vi "FG_Messen.vi"(0 "Peiker_Stepped Sweep Settings":T5={"Input Settings"={"IEPE min time to settle [s]"=0.0, "Responce Channel Settings"={"DSA response channel settings"={"coupling"=10045, "enable IEPE excitation"=FALSE, "IEPE current [mA]"=4.0}, "response channel info"={"sensor sensitivity"=1000.0, "engineering units"=1, "dB reference"=1.0, "custom label"="EU", "weighting filter"=0, "pregain"=0.0}, "AI response settings"={"response channel"="SOUNDACQ/ai1", "max value [V]"=10.0, "min value [V]"=-10.0, "terminal configuration"=-1}}, "Stimulus Channel Settings"={"AI stimulus settings"={"stimulus channel"="SOUNDACQ/ai0", "max value [V]"=2.0, "min value [V]"=-2.0, "terminal configuration"=-1}, "DSA stimulus channel settings"={"coupling"=10045, "enable IEPE excitation"=TRUE, "IEPE current [mA]"=4.0}, "stimulus channel info"={"sensor sensitivity"=11.4, "engineering units"=2, "dB reference"=2e-05, "custom label"="EU", "weighting filter"=0, "pregain"=0.0}}}, "Output Settings"={"AO source settings"={"excitation channel"="SOUNDACQ/ao0", "max value [V]"=10.0, "min value [V]"=-10.0, "terminal configuration"=-1}}} {"Output Settings"."AO source settings"."terminal configuration" items=["Default"=-1, "RSE"=10083, "Differential"=10106, "Pseudodifferential"=12529]; "Output Settings"."AO source settings"."min value [V]" format="%0.2f"; "Output Settings"."AO source settings"."max value [V]" format="%0.2f"; "Input Settings"."Stimulus Channel Settings"."stimulus channel info"."pregain" format="%.2f"; "Input Settings"."Stimulus Channel Settings"."stimulus channel info"."weighting filter" items=["Linear", "A-weighting", "B-weighting", "C-weighting", "ITU-R 468-4", "Dolby", "CCITT", "C-message", "Wb", "Wc", "Wd", "We", "Wf", "Wh", "Wj", "Wk", "Wm", "AES17 20 kHz lowpass", "AES17 40 kHz lowpass", "AES17 20 kHz highpass", "AES17 40 kHz highpass"]; "Input Settings"."Stimulus Channel Settings"."stimulus channel info"."dB reference" format="%^.1e"; "Input Settings"."Stimulus Channel Settings"."stimulus channel info"."engineering units" items=["custom..."=0, "V"=1, "A"=21, "C"=30, "pC"=31, "s"=32, "-"=29, "Pa"=2, "N"=20, "g"=3, "m/s^2"=4, "m/s"=5, "m"=6, "mm/s"=12, "mm"=13, "micron/s"=14, "micron"=15, "in/s^2"=7, "in/s"=8, "in"=9, "mil/s"=10, "mil"=11, "rad/s^2"=16, "rad/s"=17, "rad"=18, "deg/s^2"=26, "deg/s"=27, "deg"=28, "RPM"=22, "cycle/s^2"=23, "Hz"=24, "cycle"=25, "strain"=19]; "Input Settings"."Stimulus Channel Settings"."stimulus channel info"."sensor sensitivity" format="%#_5f"; "Input Settings"."Stimulus Channel Settings"."DSA stimulus channel settings"."IEPE current [mA]" format="%.1f"; "Input Settings"."Stimulus Channel Settings"."DSA stimulus channel settings"."coupling" items=["AC"=10045, "DC"=10050, "GND"=10066]; "Input Settings"."Stimulus Channel Settings"."AI stimulus settings"."terminal configuration" items=["Default"=-1, "RSE"=10083, "NRSE"=10078, "Differential"=10106, "Pseudodifferential"=12529]; "Input Settings"."Stimulus Channel Settings"."AI stimulus settings"."min value [V]" format="%.2f"; "Input Settings"."Stimulus Channel Settings"."AI stimulus settings"."max value [V]" format="%.2f"; "Input Settings"."Responce Channel Settings"."AI response settings"."terminal configuration" items=["Default"=-1, "RSE"=10083, "NRSE"=10078, "Differential"=10106, "Pseudodifferential"=12529]; "Input Settings"."Responce Channel Settings"."AI response settings"."min value [V]" format="%.2f"; "Input Settings"."Responce Channel Settings"."AI response settings"."max value [V]" format="%.2f"; "Input Settings"."Responce Channel Settings"."response channel info"."pregain" format="%.2f"; "Input Settings"."Responce Channel Settings"."response channel info"."weighting filter" items=["Linear", "A-weighting", "B-weighting", "C-weighting", "ITU-R 468-4", "Dolby", "CCITT", "C-message", "Wb", "Wc", "Wd", "We", "Wf", "Wh", "Wj", "Wk", "Wm", "AES17 20 kHz lowpass", "AES17 40 kHz lowpass", "AES17 20 kHz highpass", "AES17 40 kHz highpass"]; "Input Settings"."Responce Channel Settings"."response channel info"."dB reference" format="%^.1e"; "Input Settings"."Responce Channel Settings"."response channel info"."engineering units" items=["custom..."=0, "V"=1, "A"=21, "C"=30, "pC"=31, "s"=32, "-"=29, "Pa"=2, "N"=20, "g"=3, "m/s^2"=4, "m/s"=5, "m"=6, "mm/s"=12, "mm"=13, "micron/s"=14, "micron"=15, "in/s^2"=7, "in/s"=8, "in"=9, "mil/s"=10, "mil"=11, "rad/s^2"=16, "rad/s"=17, "rad"=18, "deg/s^2"=26, "deg/s"=27, "deg"=28, "RPM"=22, "cycle/s^2"=23, "Hz"=24, "cycle"=25, "strain"=19]; "Input Settings"."Responce Channel Settings"."response channel info"."sensor sensitivity" format="%#_5f"; "Input Settings"."Responce Channel Settings"."DSA response channel settings"."IEPE current [mA]" format="%.1f"; "Input Settings"."Responce Channel Settings"."DSA response channel settings"."coupling" items=["AC"=10045, "DC"=10050, "GND"=10066]; "Input Settings"."IEPE min time to settle [s]" format="%.1f"}, 1 "settling time":T11={"settle time [s]"=0.03, "settle cycles"=5} {"settle time [s]" format="%.2p"}, 2 "FrequencyList Output Level (dBSPL)":dbl=94.0, 5 "frequency list Input":T4(array[cluster])=[{"frequency [Hz]"=103.0, "amplitude [V]"=0.09342446715491094}] {"amplitude [V]" format="%.6f"; "frequency [Hz]" format="%.2f"}, 9 "true=mehrfach Messen":bool, 11 "error in (no error)":errorcluster, 12 "FrequencyList Input Level (dBSPL)":dbl=94.0, 13 "integration time":T10={"integration time [s]"=0.03, "integration cycles"=5} {"integration cycles" min=2; "integration time [s]" format="%.2p"}) -> (3 "Fundamental-Response":T1(graph), 4 "THD-Response":cluster{"frequency":dbl[], "THD":dbl[]}(graph), 6 "Harmonics-Response":cluster{"frequency":dbl[], "distortion":dbl[]}[](graph), 8 "Fundamental-Response dB berechnet":T3(graph) caption="Fundamental-Response dB berechnet aus THD-Modul", 10 "fundamental amplitude":T1, 14 "Stimulus Level":cluster{"frequency":dbl[], "magnitude":dbl[]}(graph), 15 "error out":errorcluster={"status"=FALSE, "code"=0, "source"="\r\n"})   [LabVIEW 2018]
doc: "Das VI dient dem Messen eines Frequenzgangs. \nDieser kann verwendet werden um den Speaker abzugleichen.\nEin abweichender Pegel darf erst angegeben werden, wenn ein Speakerabgleich auf 94 dBSpl erfolgt ist.\n\nDie 94dB Spannungswerte werden dann auf den gewünschten Pegel umgerechnet."
uses:
  Peiker_Stepped Sweep Settings.ctl
  <vilib>/addons/_NISVFA/_Shared subVIs/Controls/svc_DSA Channel Settings.ctl
  <vilib>/addons/_NISVFA/_Shared subVIs/Controls/svc_Channel Info.ctl
  <vilib>/addons/_NISVFA/_Shared subVIs/Controls/svc_Engineering Units Text Ring.ctl
  <vilib>/addons/_NISVFA/_Shared subVIs/Controls/svc_Weighting Filter Text Ring.ctl
  <vilib>/addons/Sound and Vibration/svt_Swept Sine/SVT Initialize Swept Sine (DAQmx) (1 AO, 2 AI).vi
  <vilib>/addons/_NISVFA/_Baseband FFT/SVFA Power Spectrum (N Ch).vi
  <vilib>/addons/Sound and Vibration/svt_Swept Sine/SoundVib_SweptSine.lvlib
panel:
  out "Waveform Graph 4":waveform(dbl)[](graph)
  in  "Tab Control":T2(tab)
  out "Waveform Graph 2":waveform(dbl)[](graph)
  in  "Messkurve":dbl min=0.0 max=28.0
  out "Block Duration":waveform(dbl)[](graph)
  in  "stop":bool
  in  "Enable this Diagramm":bool
  out "Waveform Graph 3":cluster{"f0":dbl, "df":dbl, "magnitude":dbl[]}[](graph)
  out "Response Level":cluster{"frequency":dbl[], "magnitude":dbl[]}(graph)
  out "THD":cluster{"frequency":dbl[], "THD":dbl[]}={"frequency"=[103.0], "THD"=[0.2630754420190896]} {"THD" format="%.2f"; "frequency" format="%.2f"}
  out "Waveform Graph":cluster{"f0":dbl, "df":dbl, "magnitude":dbl[]}[](graph)
  out "FrequencyList Output Level":T4(graph)
  in  "Anzahl der Messungen bei einer Frequenz":i32=10
  in  "block duration [ms]":dbl=30.0
  in  "sample rate [Hz]":dbl=50000.0
  out "status":T12 {"% complete" format="%.2f"; "current processed frequency" format="%.2f"; "current source frequency" format="%.2f"; "elapsed time [s]" format="%.2f"}
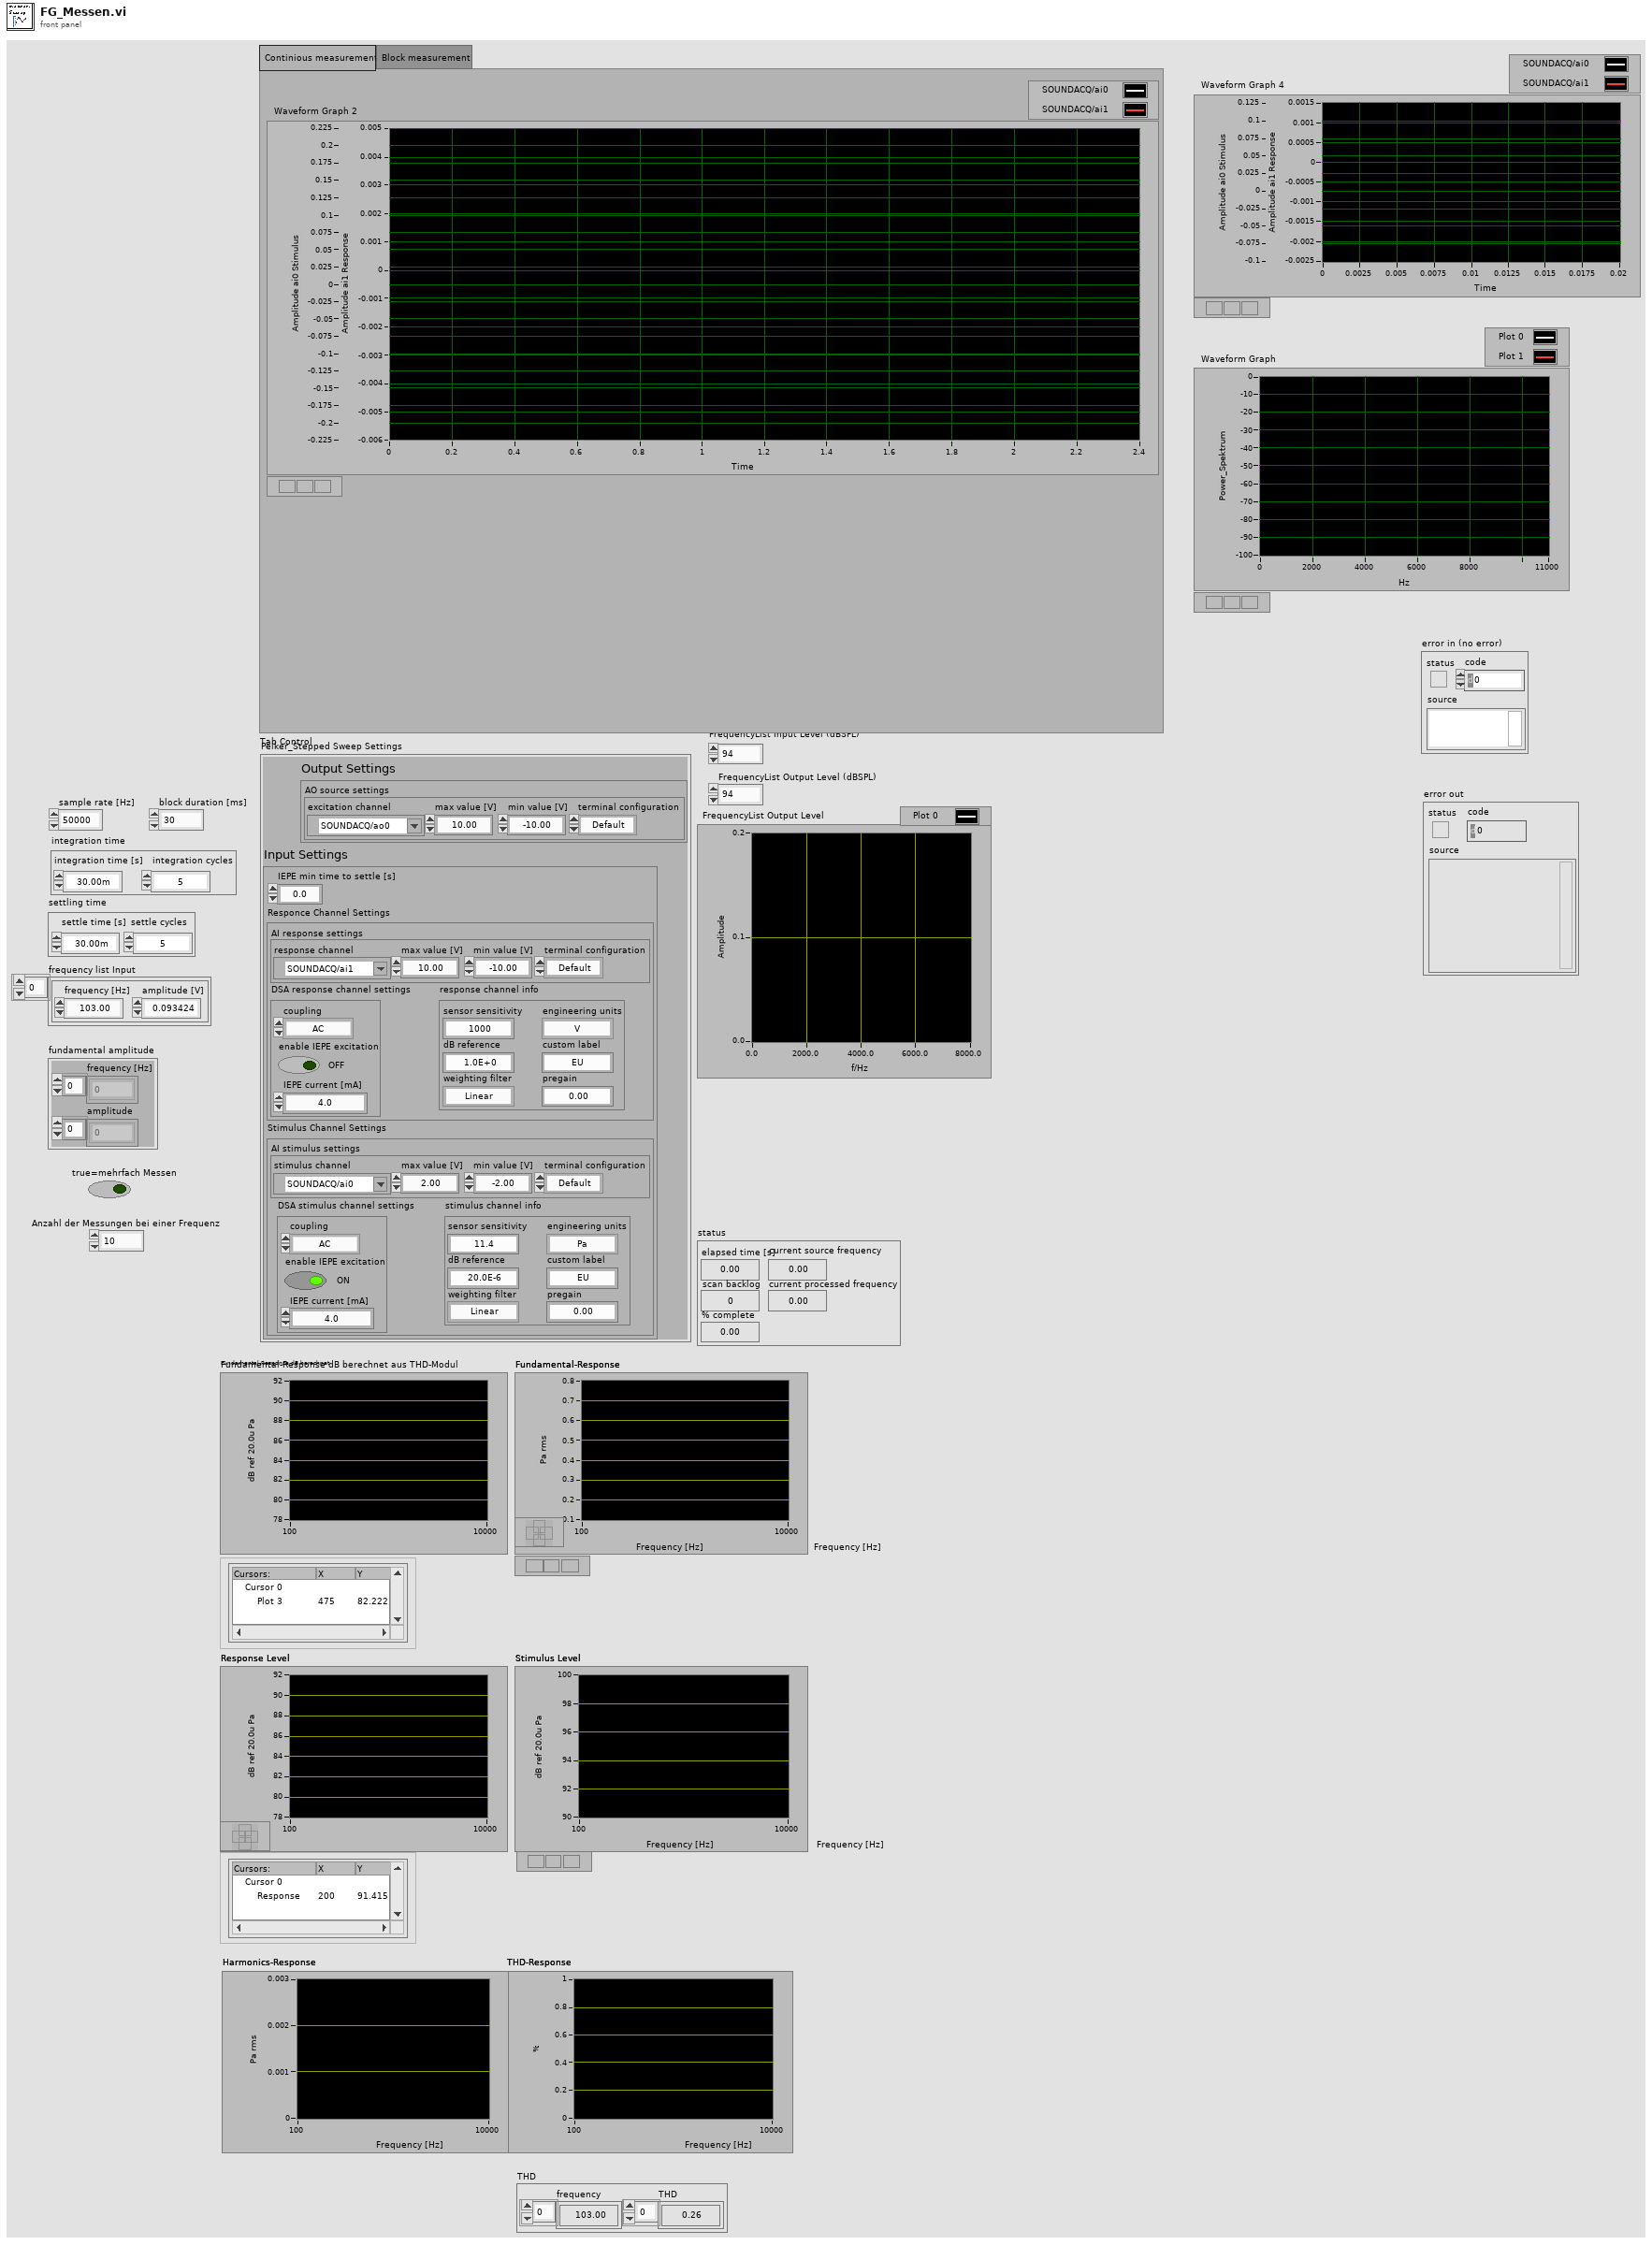
[diagram p1: front panel]
types:
  T1 = cluster{"frequency [Hz]":dbl[], "amplitude":dbl[]}
  T2 = enum32{"Continious measurement", "Block measurement"}
  T3 = cluster{"frequency [Hz]":dbl[], "amplitude":dbl[]}[]
  T4 = cluster{"frequency [Hz]":dbl, "amplitude [V]":dbl}[]
  T5 = typedef "Peiker_Stepped Sweep Settings.ctl" = cluster{"Input Settings":cluster{"IEPE min time to settle [s]":dbl, "Responce Channel Settings":cluster{"DSA response channel settings":T6, "response channel info":T7, "AI response settings":cluster{"response channel":tag, "max value [V]":dbl, "min value [V]":dbl, "terminal configuration":i32}}, "Stimulus Channel Settings":cluster{"AI stimulus settings":cluster{"stimulus channel":tag, "max value [V]":dbl, "min value [V]":dbl, "terminal configuration":i32}, "DSA stimulus channel settings":T6, "stimulus channel info":T7}}, "Output Settings":cluster{"AO source settings":cluster{"excitation channel":tag, "max value [V]":dbl, "min value [V]":dbl, "terminal configuration":i32}}}
  T6 = typedef "svc_DSA Channel Settings.ctl" = cluster{"coupling":i32, "enable IEPE excitation":bool, "IEPE current [mA]":dbl}
  T7 = typedef "svc_Channel Info.ctl" = cluster{"sensor sensitivity":dbl, "engineering units":T8, "dB reference":dbl, "custom label":string, "weighting filter":T9, "pregain":dbl}
  T8 = typedef "svc_Engineering Units Text Ring.ctl" = u16
  T9 = typedef "svc_Weighting Filter Text Ring.ctl" = u16
  T10 = cluster{"integration time [s]":dbl, "integration cycles":i32}
  T11 = cluster{"settle time [s]":dbl, "settle cycles":i32}
  T12 = cluster{"elapsed time [s]":dbl, "scan backlog":u32, "current source frequency":dbl, "current processed frequency":dbl, "% complete":dbl}
  T13 = cluster{"excitation channel":tag, "max value [V]":dbl, "min value [V]":dbl, "terminal configuration":i32}
  T14 = cluster{"stimulus channel":tag, "max value [V]":dbl, "min value [V]":dbl, "terminal configuration":i32}
  T15 = cluster{"response channel":tag, "max value [V]":dbl, "min value [V]":dbl, "terminal configuration":i32}
  T16 = typedef "SoundVib_SweptSine.lvlib/sv_Swept Sine Task.ctl" = cluster{"source settings":cluster{"AO task name":refnum<k21>, "source":cluster{"AO physical channel":tag}[]}, "stimulus settings":cluster{"stimulus task name":refnum<k21>, "stimulus":cluster{"stimulus physical channel":tag, "channel info":T7}[]}, "response(s) settings":cluster{"response task name":refnum<k21>, "response":cluster{"response physical channel":tag, "channel info":T7}[]}, "measurement settings":cluster{"AI sampling frequency":dbl, "AO sampling frequency":dbl, "AI block size":i32, "AO block Size":i32, "block duration [ms]":dbl, "number of AI channels":i32, "device propagation delay [samples]":dbl, "total propagation time [samples]":dbl, "DUT propagation time [ms]":dbl}, "linlog":enum16{"linear", "log"}, "repeat":enum16{"off", "on"}, "frequency list":dbl[], "amplitude list":dbl[], "settling time":cluster{"settle time":dbl, "settle cycles":i32}, "integration time":cluster{"integration time":dbl, "integration cycles":i32}, "frequencies indices":cluster{"AI freq index":i32, "AO freq index":i32}, "read marks":cluster{"write index":u32, "read index":u32, "freq start index":u32, "freq stop index":u32, "# extracted":u32, "buffer type":enum16{"Invalid buffer", "Intermediate buffer", "Final buffer"}, "read/write indices":cluster{"settle time index":u32, "integration time index":u32}[], "AO index":i32, "AI index":i32, "settled":bool, "integration done":bool}, "harmonic settings":cluster{"maximum THD harmonic":u32, "harmonic mapping":u32[], "units":cluster{"THD unit":enum16{"dB", "%"}, "nth harmonic unit":enum16{"dB", "%"}, "SINAD unit":enum16{"dB", "%"}, "THD+N unit":enum16{"dB", "%"}}}, "auto resolution settings":cluster{"auto max step":i32, "slow threshold db":dbl, "fast threshold db":dbl}, "auto level settings":cluster{"auto level enable":bool, "auto level channel":u8, "ideal ref":sgl, "max level":sgl, "ref upper deviation db":sgl, "ref lower deviation db":sgl}, "offset":dbl, "ramping rate":dbl, "phase":dbl, "initialize":bool}
  T17 = enum16{"EU rms", "EU peak", "EU peak-peak", "dB ref fund"}
  T18 = cluster{"THD units":enum16{"dB", "linear ratio", "%"}, "harmonic component amplitude units":enum16{"EU rms", "EU peak", "EU peak-peak", "dB ref fund"}, "fundamental amplitude units":enum16{"EU rms", "EU peak", "EU peak-peak"}}
  T19 = typedef "SoundVib_SweptSine.lvlib/sv_Swept Sine Measurements.ctl" = cluster{"RMS stimulus":dbl[], "RMS response":dbl[], "Re [stimulus]":dbl[], "Im [stimulus]":dbl[], "Re [response]":dbl[], "Im [response]":dbl[], "THD":dbl[], "Harm[]":dbl[][], "scaled response magnitude":dbl[]}
  T20 = cluster{"THD unit label":string, "harmonic component amplitudes unit label":string, "fundamental amplitude unit label":string}
  T21 = cluster{"response physical channel":tag, "channel info":T7}[]
  T22 = cluster{"response physical channel":tag, "channel info":T7}
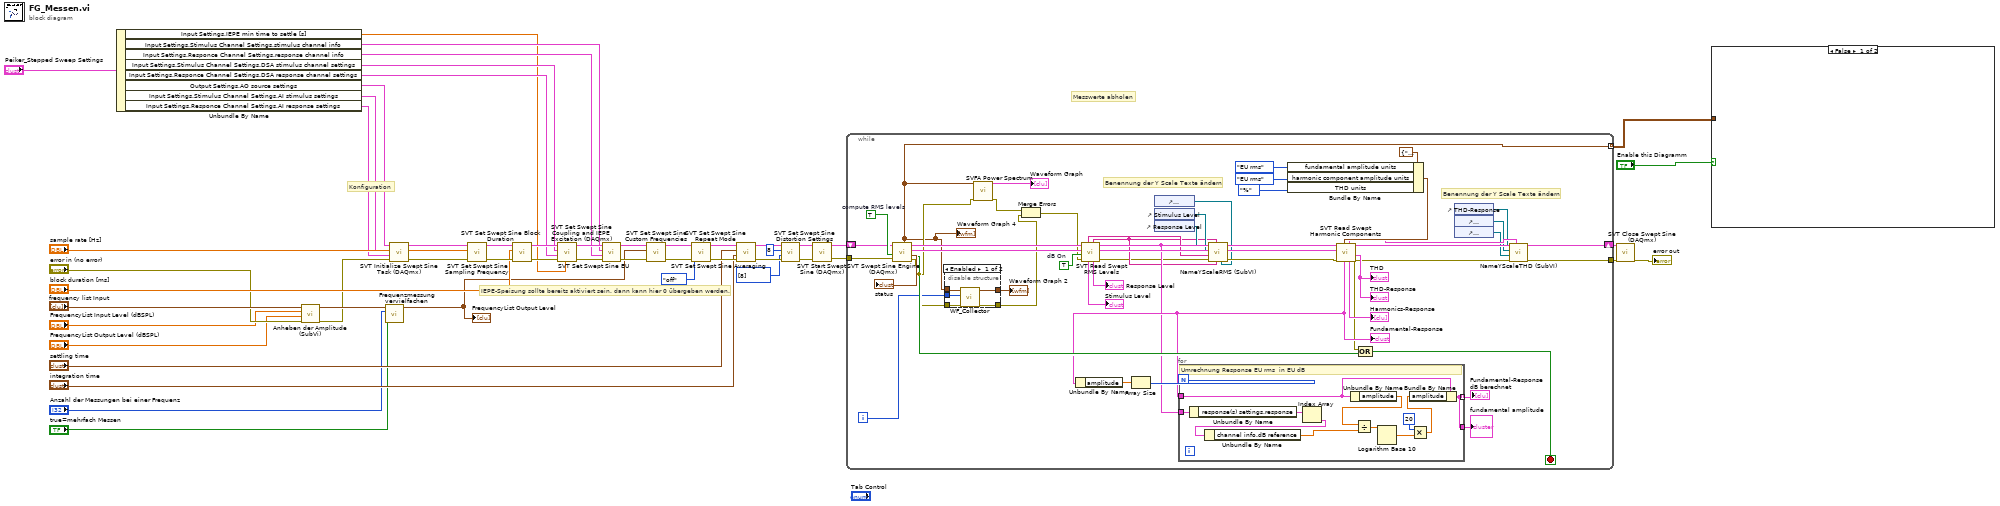
[diagram p0: block diagram]
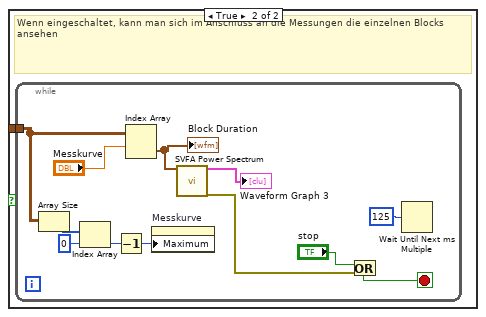
[diagram p2: hidden frame]
diagram:
  # "IEPE-Speisung sollte bereits aktiviert sein. dann kann hier 0 übergeben werden."
  # "Messwerte abholen"
  # "Konfiguration"
  n1 = Unbundle By Name("Peiker_Stepped Sweep Settings") -> ("Input Settings.IEPE min time to settle [s]"=w15:dbl, "Input Settings.Stimulus Channel Settings.stimulus channel info"=w20:T7, "Input Settings.Responce Channel Settings.response channel info"=w21:T7, "Input Settings.Stimulus Channel Settings.DSA stimulus channel settings"=w22:T6, "Input Settings.Responce Channel Settings.DSA response channel settings"=w23:T6, "Output Settings.AO source settings"=w29:T13, "Input Settings.Stimulus Channel Settings.AI stimulus settings"=w17:T14, "Input Settings.Responce Channel Settings.AI response settings"=w16:T15)
  n2 = call "Anheben der Amplitude (SubVi).vi"("error In"="error in (no error)", "FrequencyList Output Level (calc)"="FrequencyList Output Level (dBSPL)", "FrequencyList Input Level"="FrequencyList Input Level (dBSPL)", "custom frequency list Input"="frequency list Input") -> ("error Out"=w7:errorcluster, "custom frequency list Output"=w10:T4)  [unwired: 5 in, 1 out]
  n3 = call "Frequenzmessung vervielfachen.vi"("true=mehrfach Messen"="true=mehrfach Messen", "Anzahl der Messungen bei einer Frequenz"="Anzahl der Messungen bei einer Frequenz", "Eingang"=w10) -> ("Ausgang"=w12:T4)  [unwired: 8 in]
  "FrequencyList Output Level" <- w12
  n4 = call-poly <vilib>:"SVT Initialize Swept Sine Task (DAQmx).vi"("error in (no error)"=w7, "AI response settings"=w16, "AI stimulus settings"=w17, "AO source settings"=w29) -> ("error out"=w2:errorcluster, "swept sine task out"=w1:T16)  [unwired: 6 in]
  n5 = call <vilib>:"SVT Set Swept Sine Sampling Frequency.vi"("error in (no error)"=w2, "sampling frequency\n[samples/s]"="sample rate [Hz]", "swept sine task in"=w1) -> ("error out"=w34:errorcluster, "swept sine task out"=w35:T16)  [unwired: 7 in]
  n6 = call <vilib>:"SVT Set Swept Sine Block Duration.vi"("error in (no error)"=w34, "block duration [ms]"="block duration [ms]", "swept sine task in"=w35) -> ("error out"=w50:errorcluster, "swept sine task out"=w49:T16)  [unwired: 7 in]
  n7 = call <vilib>:"SVT Set Swept Sine Coupling and IEPE Excitation (DAQmx).vi"("time to settle [s]"=w15, "error in (no error)"=w50, "DSA response channel settings"=w23, "DSA stimulus channel settings"=w22, "swept sine task in"=w49) -> ("error out"=w47:errorcluster, "swept sine task out"=w48:T16)  [unwired: 5 in]
  n8 = call <vilib>:"SVT Set Swept Sine EU.vi"("error in (no error)"=w47, "response channel info"=w21, "stimulus channel info"=w20, "swept sine task in"=w48) -> ("error out"=w46:errorcluster, "swept sine task out"=w45:T16)  [unwired: 6 in]
  n9 = call <vilib>:"SVT Set Swept Sine Custom Frequencies.vi"("error in (no error)"=w46, "custom frequency list"=w12, "swept sine task in"=w45) -> ("error out"=w32:errorcluster, "swept sine task out"=w33:T16)  [unwired: 7 in]
  n10 = call <vilib>:"SVT Set Swept Sine Repeat Mode.vi"("error in (no error)"=w32, "repeat"=enum16{"off", "on"}."off", "swept sine task in"=w33) -> ("error out"=w44:errorcluster, "swept sine task out"=w43:T16)  [unwired: 7 in]
  n11 = call <vilib>:"SVT Set Swept Sine Averaging.vi"("error in (no error)"=w44, "integration time"="integration time", "settling time"="settling time", "swept sine task in"=w43) -> ("error out"=w41:errorcluster, "swept sine task out"=w42:T16)  [unwired: 6 in]
  n12 = call <vilib>:"SVT Set Swept Sine Distortion Settings.vi"("error in (no error)"=w41, "harmonics to visualize"=u32[] [8], "maximum harmonic"=u32 8, "swept sine task in"=w42) -> ("error out"=w39:errorcluster, "swept sine task out"=w40:T16)  [unwired: 6 in]
  n13 = call <vilib>:"SVT Start Swept Sine (DAQmx).vi"("error in (no error)"=w39, "swept sine task in"=w40) -> ("error out"=w38:errorcluster, "swept sine task out"=w36:T16)  [unwired: 8 in]
  n14 = while {
    tunnel: w38 -> [w91]
    tunnel: [w60] -> w37
    shift-right: [w88] -> w9
    shift-left: w36 -> [w87]
    tunnel: [w52] -> w4 mode=indexing
    i -> [w57]
    stop <- w90 stop-if-true
    w94 = TRUE  # dB On
    w96 = TRUE  # compute RMS levels
    # "Benennung der Y Scale Texte ändern"
    # "Benennung der Y Scale Texte ändern"
    n15 = call <vilib>:"SVT Swept Sine Engine (DAQmx).vi"("error in (no error)"=w91, "compute RMS levels (F)"=w96, "swept sine task in"=w87) -> ("error out"=w56:errorcluster, "status"=→"status":T12, "swept sine measurements"=w76:T19, "swept sine task out"=w95:T16, "sweep done"=w89:bool, "waveform data [V]"=w52:waveform(dbl)[])  [unwired: 3 in]
    "Waveform Graph 4" <- w52
    n16 = disable-structure shown="Enabled" {
      disable-tunnel: w52 -> [w102 w103]
      disable-tunnel: w57 -> [w101 _]
      disable-tunnel: w56 -> [w100 w104]
      disable-tunnel: [w99 w104] -> w54
      disable-tunnel: [w98 w103] -> w58
      frame Enabled {
        n17 = call "WF_Collector.vi"("error in (no error)"=w100, "LoopCounter"=w101, "waveform data ClusterIn"=w102) -> ("error out"=w99:errorcluster, "waveform data ClusterOut"=w98:waveform(dbl)[])  [unwired: 7 in]
      }
      frame Disabled {
      }
    }
    "Waveform Graph 2" <- w58
    n18 = call-poly <vilib>:"SVFA Power Spectrum.vi"("scaled signals [EU]"=w52, "error in (no error)"=w56) -> ("power spectra [dB EU]"=→"Waveform Graph":cluster{"f0":dbl, "df":dbl, "magnitude":dbl[]}[], "error out"=w55:errorcluster)  [unwired: 12 in, 4 out]
    n19 = Merge Errors(w55, w54) -> (w53:errorcluster)
    n20 = call <vilib>:"SVT Read Swept RMS Levels.vi"("error in (no error)"=w53, "dB On (T)"=w94, "swept sine measurements"=w76, "swept sine task in"=w95) -> ("error out"=w59:errorcluster, "dup swept sine measurements"=w73:T19, "swept sine task out"=w72:T16, "RMS level (response)"=→"Response Level":cluster{"frequency":dbl[], "magnitude":dbl[]}, "response unit label"=w62:string, "RMS level (stimulus)"=→"Stimulus Level":cluster{"frequency":dbl[], "magnitude":dbl[]}, "stimulus unit label"=w65:string)  [unwired: 1 in]
    n21 = control-ref of="Fundamental-Response dB berechnet"() -> (w61:refnum<vi>)
    n22 = control-ref of="Stimulus Level"() -> (w63:refnum<vi>)
    n23 = control-ref of="Response Level"() -> (w64:refnum<vi>)
    n24 = call "NameYScaleRMS (SubVI).vi"("XYGraph in 2"=w61, "response unit label 2"=w62, "response unit label"=w62, "error in (no error)"=w59, "stimulus unit label"=w65, "XYGraph Refnum in"=w63, "XYGraph in"=w64) -> ("error out"=w66:errorcluster)  [unwired: 4 in]
    n25 = Bundle By Name(cluster=T18 {"THD units"=enum."dB", "harmonic component amplitude units"=enum."EU rms", "fundamental amplitude units"=enum."EU rms"} ("output cluster"), "fundamental amplitude units"=enum16{"EU rms", "EU peak", "EU peak-peak"}."EU rms", "harmonic component amplitude units"=T17."EU rms", "THD units"=enum16{"dB", "linear ratio", "%"}."%") -> (w81:T18)
    n26 = call <vilib>:"SVT Read Swept Harmonic Components.vi"("desired units"=w81, "error in (no error)"=w66, "swept sine measurements"=w73, "swept sine task in"=w72) -> ("error out"=w71:errorcluster, "THD"=→"THD-Response" →"THD":cluster{"frequency":dbl[], "THD":dbl[]}, "swept sine task out"=w88:T16, "harmonic components"=→"Harmonics-Response":cluster{"frequency":dbl[], "distortion":dbl[]}[], "unit labels"=w70:T20, "fundamental amplitude"=w77:T1)  [unwired: 1 in, 1 out]
    "Fundamental-Response" <- w77
    n27 = Unbundle By Name(w77) -> ("amplitude"=w84:dbl[])
    n28 = Array Size(array=w84) -> (size(s)=w83:i32)
    n29 = for {
      N: w83 -> [_]
      tunnel: w77 -> [w111]
      tunnel: [w105] -> w85 mode=indexing
      tunnel: w72 -> [w108]
      tunnel: [w105] -> w51
      # "Umrechnung Response EU rms  in EU dB"
      n30 = Unbundle By Name(w108) -> ("response(s) settings.response"=w107:T21)
      n31 = Index Array(array=w107) -> (element=w109:T22)  [unwired: 1 in]
      n32 = Unbundle By Name(w109) -> ("channel info.dB reference"=w106:dbl)
      n33 = Unbundle By Name(w111) -> ("amplitude"=w114:dbl[])
      n34 = Divide(x=w114, y=w106) -> (x/y=w115:dbl[])
      n35 = Logarithm Base 10(1:w115) -> (0:w112:dbl[])
      n36 = Multiply(x=20, y=w112) -> (x*y=w110:dbl[])
      n37 = Bundle By Name(cluster=w111, "amplitude"=w110) -> (w105:T1)
    }
    "Fundamental-Response dB berechnet" <- w85
    "fundamental amplitude" <- w51
    n38 = Compound Arithmetic op=OR(w71, w89) -> (w90:bool)
    n39 = control-ref of="THD-Response"() -> (w69:refnum<vi>)
    n40 = control-ref of="Harmonics-Response"() -> (w68:refnum<vi>)
    n41 = control-ref of="Fundamental-Response"() -> (w67:refnum<vi>)
    n42 = call "NameYScaleTHD (SubVI).vi"("unit labels"=w70, "error in (no error)"=w71, "XYGraph Refnum 3"=w67, "XYGraph Refnum in"=w68, "XYGraph in"=w69) -> ("error out"=w60:errorcluster)  [unwired: 6 in]
  }
  n43 = call <vilib>:"SVT Close Swept Sine (DAQmx).vi"("error in (no error)"=w37, "swept sine task in"=w9) -> ("error out"=→"error out":errorcluster)  [unwired: 9 in]
  n44 = case shown="False" "Enable this Diagramm" {
    tunnel: w4 -> [_ w116]
    frame False {
    }
    frame True {
      # "Wenn eingeschaltet, kann man sich im Anschluss an die Messungen die einzelnen Blocks ansehen"
      n45 = while {
        tunnel: w116 -> [w119]
        stop <- w118 stop-if-true
        n46 = Array Size(array=w119) -> (size(s)=w123:i32[])
        n47 = Index Array(array=w123, index=0) -> (element=w121:i32)
        n48 = Decrement(x=w121) -> (x-1=w120:i32)
        n49 = Index Array(array=w119, index (row)="Messkurve") -> (element=w125:waveform(dbl)[])  [unwired: 1 in]
        "Block Duration" <- w125
        n50 = property on="Messkurve" class="DigNum (strict)"("Maximum"=w120) -> ()  [unwired: 2 in, 2 out]
        n51 = call-poly <vilib>:"SVFA Power Spectrum.vi"("scaled signals [EU]"=w125) -> ("power spectra [dB EU]"=→"Waveform Graph 3":cluster{"f0":dbl, "df":dbl, "magnitude":dbl[]}[], "error out"=w117:errorcluster)  [unwired: 13 in, 4 out]
        n52 = Or(x="stop", y=w117) -> (x .or. y?=w118:bool)
        n53 = Wait Until Next ms Multiple(millisecond multiple=u32 125) -> ()  [unwired: 1 out]
      }
    }
  }
